vi "MailMessage.vi"(8 "AddSubject":string, 9 "message":string, 10 "file path":path, 11 "program":string) -> ()   [LabVIEW 2012]
uses:
  <vilib>/addons/database/Connection.llb/DB Tools Open Connec (Path).vi
  <vilib>/addons/database/Connection.llb/Conn Execute.vi
  <vilib>/addons/database/Recordset.llb/Rec Fetch String Data (R).vi
  <vilib>/addons/database/Recordset.llb/Rec Destroy - Connection.vi
  <vilib>/addons/database/Recordset.llb/Rec Fetch Recordset Data (R).vi
  <vilib>/addons/database/_DB Variant To Data/Database Variant To Data.xnode
  <vilib>/addons/database/NI_Database_API.lvlib
  <vilib>/Utility/SMTP/NI_SMTPEmail.lvlib
panel:
  out "x > y?":bool
  out "error out 2":errorcluster
  in  "MIME content-type (application/octet-stream)":string="application/octet-stream"
  out "Sender":string[](array[string])
  out "Array":string[](array[string])
  out "returnMail":string
  out "Subject":string
  out "error out":errorcluster
  out "concatenated string":string
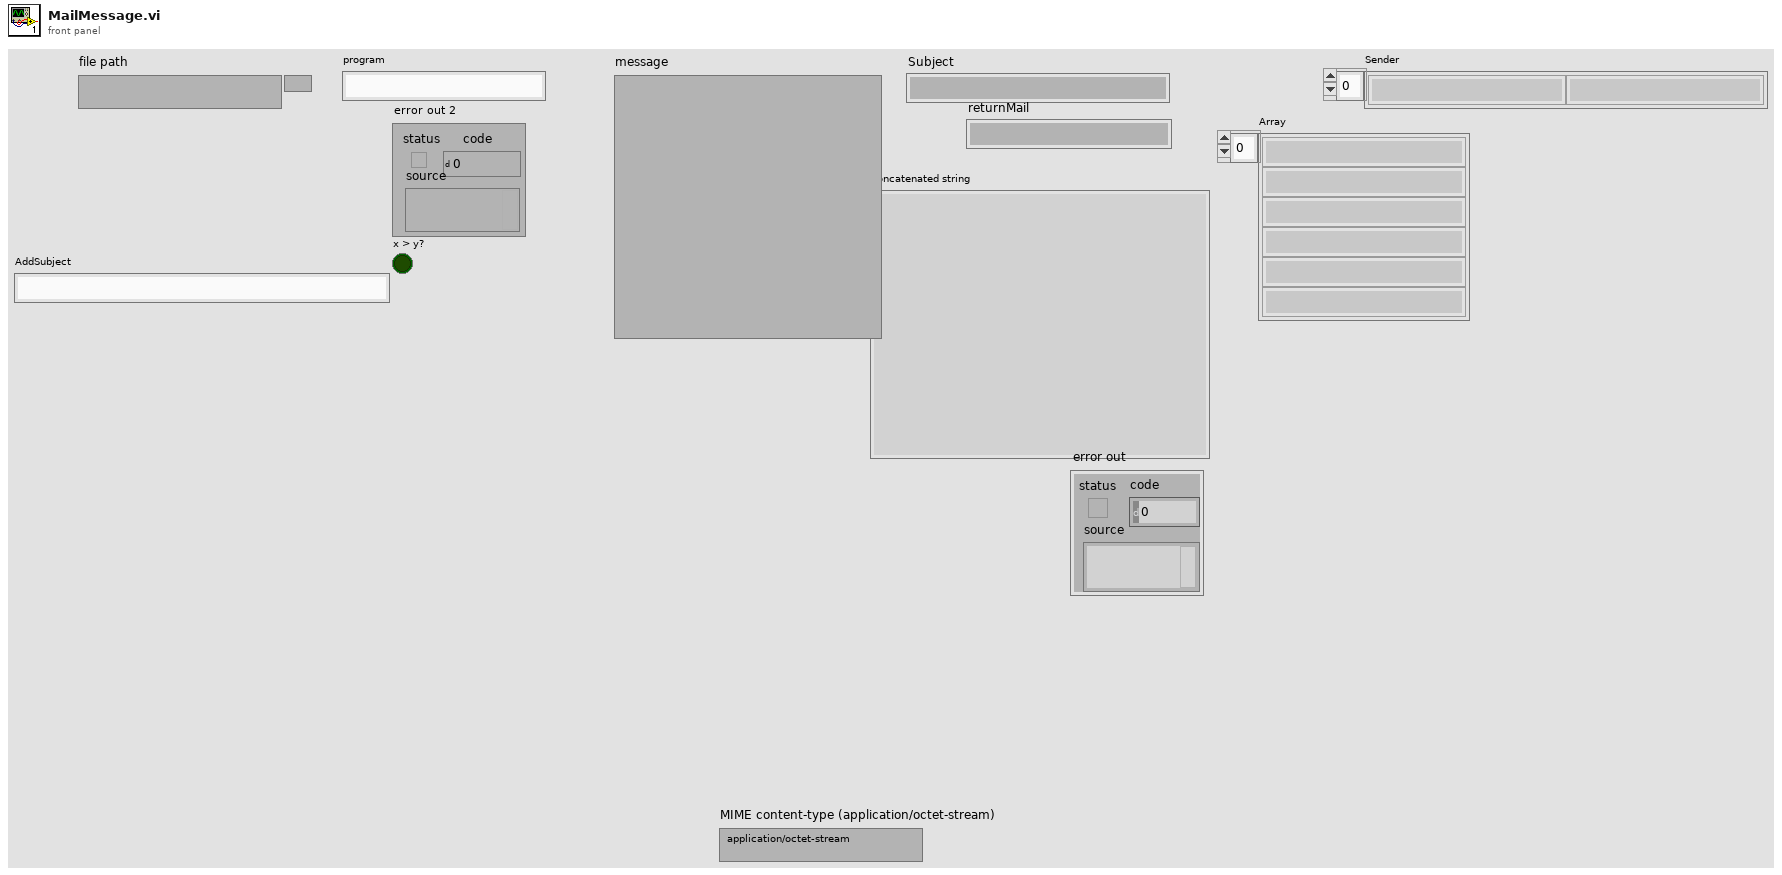
[diagram p1: front panel]
types:
  T1 = typedef "NI_Database_API.lvlib/Conn ObjectReference.ctl" = refnum<k1>
  T2 = typedef "NI_Database_API.lvlib/Rec ObjectReference.ctl" = refnum<k1>
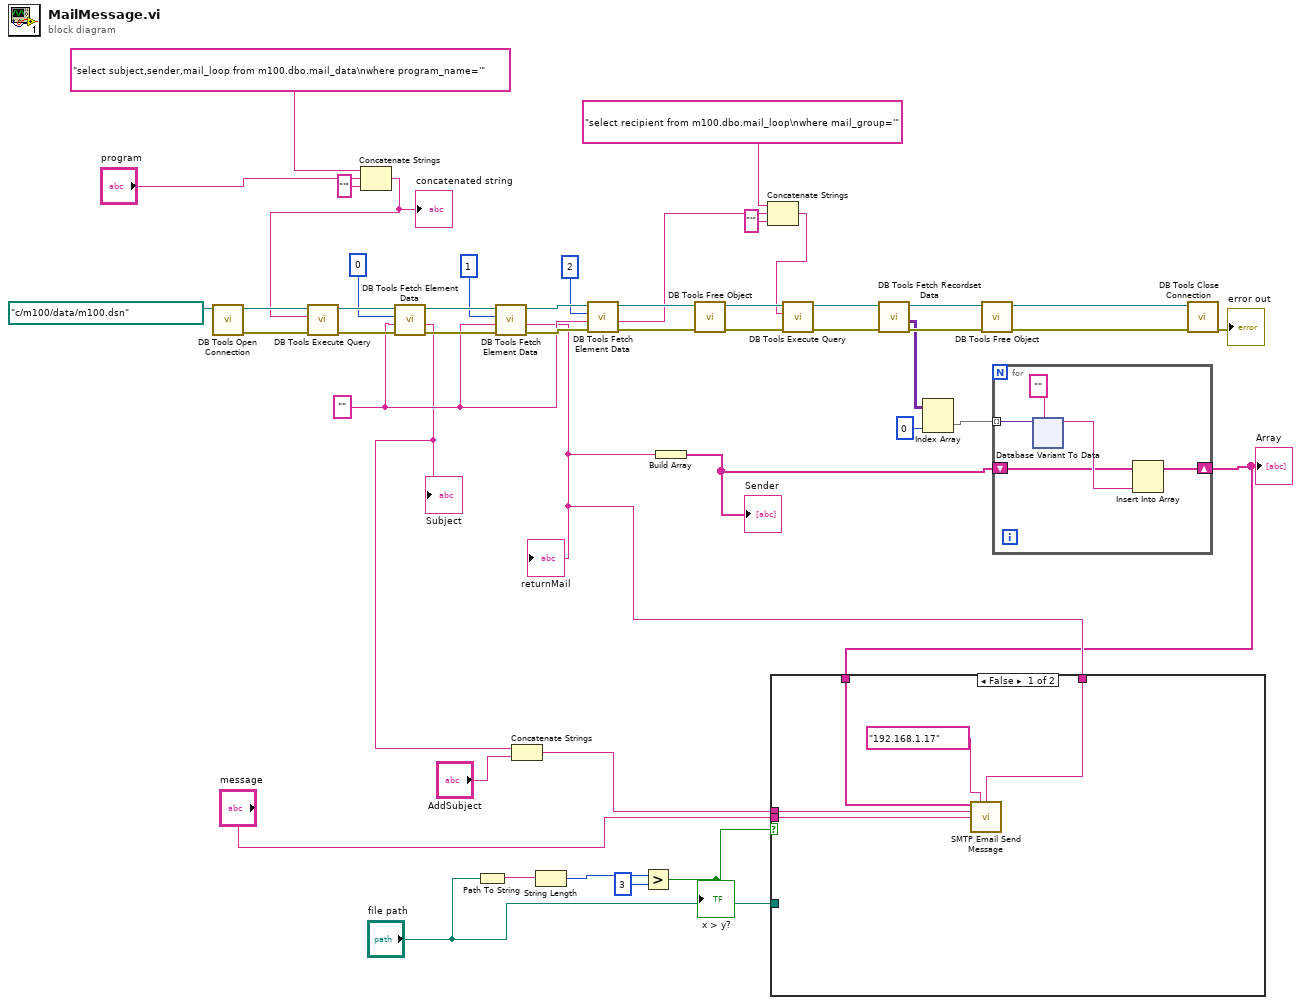
[diagram p0: block diagram]
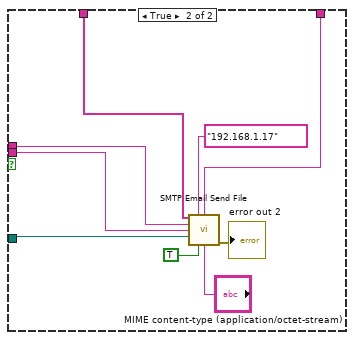
[diagram p2: hidden frame]
diagram:
  w28 = ""
  n1 = call-poly <vilib>:"DB Tools Open Connection.vi"("connection information"=path "c:/m100/data/m100.dsn") -> ("error out"=w44:errorcluster, "connection reference"=w46:T1)  [unwired: 7 in]
  n2 = Concatenate Strings("select subject,sender,mail_loop from m100.dbo.mail_data\nwhere program_name='" ("string"), "program", "'" ("string")) -> (w41:string)
  "concatenated string" <- w41
  n3 = call-poly <vilib>:"DB Tools Execute Query.vi"("error in (no error)"=w44, "SQL query"=w41, "connection reference"=w46) -> ("error out"=w43:errorcluster, "recordset reference"=w45:T2)  [unwired: 5 in]
  n4 = call-poly <vilib>:"DB Tools Fetch Element Data.vi"("error in (no error)"=w43, "type"=w28, "column index"=0, "recordset reference"=w45) -> ("error out"=w34:errorcluster, "data"=w4:string, "recordset reference out"=w37:T2)  [unwired: 3 in]
  "Subject" <- w4
  n5 = Path To String(path="file path") -> (string=w8:string)
  n6 = call-poly <vilib>:"DB Tools Fetch Element Data.vi"("error in (no error)"=w34, "type"=w28, "column index"=1, "recordset reference"=w37) -> ("error out"=w33:errorcluster, "data"=w12:string, "recordset reference out"=w36:T2)  [unwired: 3 in]
  "returnMail" <- w12
  n7 = Concatenate Strings(w4, "AddSubject") -> (w3:string)
  n8 = String Length(string=w8) -> (length=w7:i32)
  n9 = call-poly <vilib>:"DB Tools Fetch Element Data.vi"("error in (no error)"=w33, "type"=w28, "column index"=2, "recordset reference"=w36) -> ("error out"=w32:errorcluster, "data"=w18:string, "recordset reference out"=w35:T2)  [unwired: 3 in]
  n10 = Greater?(x=w7, y=3) -> (0:w5:bool)
  "x > y?" <- w5
  n11 = Build Array(w12) -> (w1:string[])
  "Sender" <- w1
  n12 = call-poly <vilib>:"DB Tools Free Object.vi"("error in (no error)"=w32, "recordset reference"=w35) -> ("error out"=w23:errorcluster, "connection reference"=w27:T1)  [unwired: 8 in]
  n13 = Concatenate Strings("select recipient from m100.dbo.mail_loop\nwhere mail_group='" ("string"), w18, "'" ("string")) -> (w16:string)
  n14 = call-poly <vilib>:"DB Tools Execute Query.vi"("error in (no error)"=w23, "SQL query"=w16, "connection reference"=w27) -> ("error out"=w22:errorcluster, "recordset reference"=w26:T2)  [unwired: 5 in]
  n15 = call-poly <vilib>:"DB Tools Fetch Recordset Data.vi"("error in (no error)"=w22, "recordset reference"=w26) -> ("error out"=w21:errorcluster, "recordset data"=w15:variant[][], "recordset reference out"=w25:T2)  [unwired: 3 in]
  n16 = Index Array(array=w15, index (col)=0 ("disabled index (col)")) -> (element=w13:variant[])  [unwired: 1 in]
  n17 = call-poly <vilib>:"DB Tools Free Object.vi"("error in (no error)"=w21, "recordset reference"=w25) -> ("error out"=w20:errorcluster, "connection reference"=w24:T1)  [unwired: 8 in]
  n18 = for {
    tunnel: w13 -> [w52] mode=indexing
    shift-right: [w49] -> w11
    shift-left: w1 -> [w48]
    n19 = xnode "Database Variant To Data"("database variant"=w52, "type"="") -> ("data"=w50:string)  [unwired: 1 in, 1 out]
    n20 = Insert Into Array(array=w48, new element=w50) -> (w49:string[])  [unwired: 1 in]
  }
  "Array" <- w11
  n21 = case shown="False" w5 {
    tunnel: w12 -> [w88 w93]
    tunnel: w11 -> [w87 w92]
    tunnel: w3 -> [w86 w95]
    tunnel: "message" -> [w85 w94]
    tunnel: "file path" -> [_ w91]
    frame False {
      n22 = call <vilib>:"SMTP Email Send Message.vi"("recipients"=w87, "mail server"="192.168.1.17", "return address"=w88, "subject ([No Subject])"=w86, "message"=w85) -> ()  [unwired: 9 in, 2 out]
    }
    frame True {
      n23 = call <vilib>:"SMTP Email Send File.vi"("recipients"=w92, "mail server"="192.168.1.17", "return address"=w93, "subject ([No Subject])"=w95, "message"=w94, "file path"=w91, "binary? (F)"=TRUE, "MIME content-type (application/octet-stream)"="MIME content-type (application/octet-stream)") -> ("error out"=→"error out 2":errorcluster)  [unwired: 6 in, 1 out]
    }
  }
  n24 = call <vilib>:"DB Tools Close Connection.vi"("error in (no error)"=w20, "connection reference"=w24) -> ("error out"=→"error out":errorcluster)  [unwired: 5 in]
